vi "Untitled 2 (SubVI).vi"(6 "input cluster in":T1 {"Image Type" items=["Grayscale (U8)", "Grayscale (U16)"]; "ROI Parameters"."Size(um)" min=0 max=255 step=0.1 format="%.2f"; "ROI Parameters"."Count" min=0 max=255 step=0.1 format="%.2f"}, 7 "Variant":variant, 8 "error in (no error)":errorcluster, 9 "reference 3":refnum<vi>, 10 "reference in":refnum<vi>, 11 "Digital in":refnum<vi>) -> (0 "error out":errorcluster, 1 "input cluster out":T1 {"Image Type" items=["Grayscale (U8)", "Grayscale (U16)"]; "ROI Parameters"."Size(um)" min=0 max=255 step=0.1 format="%.2f"; "ROI Parameters"."Count" min=0 max=255 step=0.1 format="%.2f"}, 2 "Address Var":variant, 3 "Error Var":variant)   [LabVIEW 2023, in "Camera_Controller.lvlib" / "Camera_Controller.lvclass"]
uses:
  Camera_Controller.lvclass
  Camera_Controller.lvclass/Camera_Controller.ctl
  <userlib>/_OpenG.lib/lvdata/lvdata.llb/openg_variant.lvlib
  <vilib>/vision/Image Controls.llb/IMAQ Image.ctl
  typedefs/Image Type.ctl
  typedefs/typedefs.lvlib
  typedefs/ImageProcessingParameters.ctl
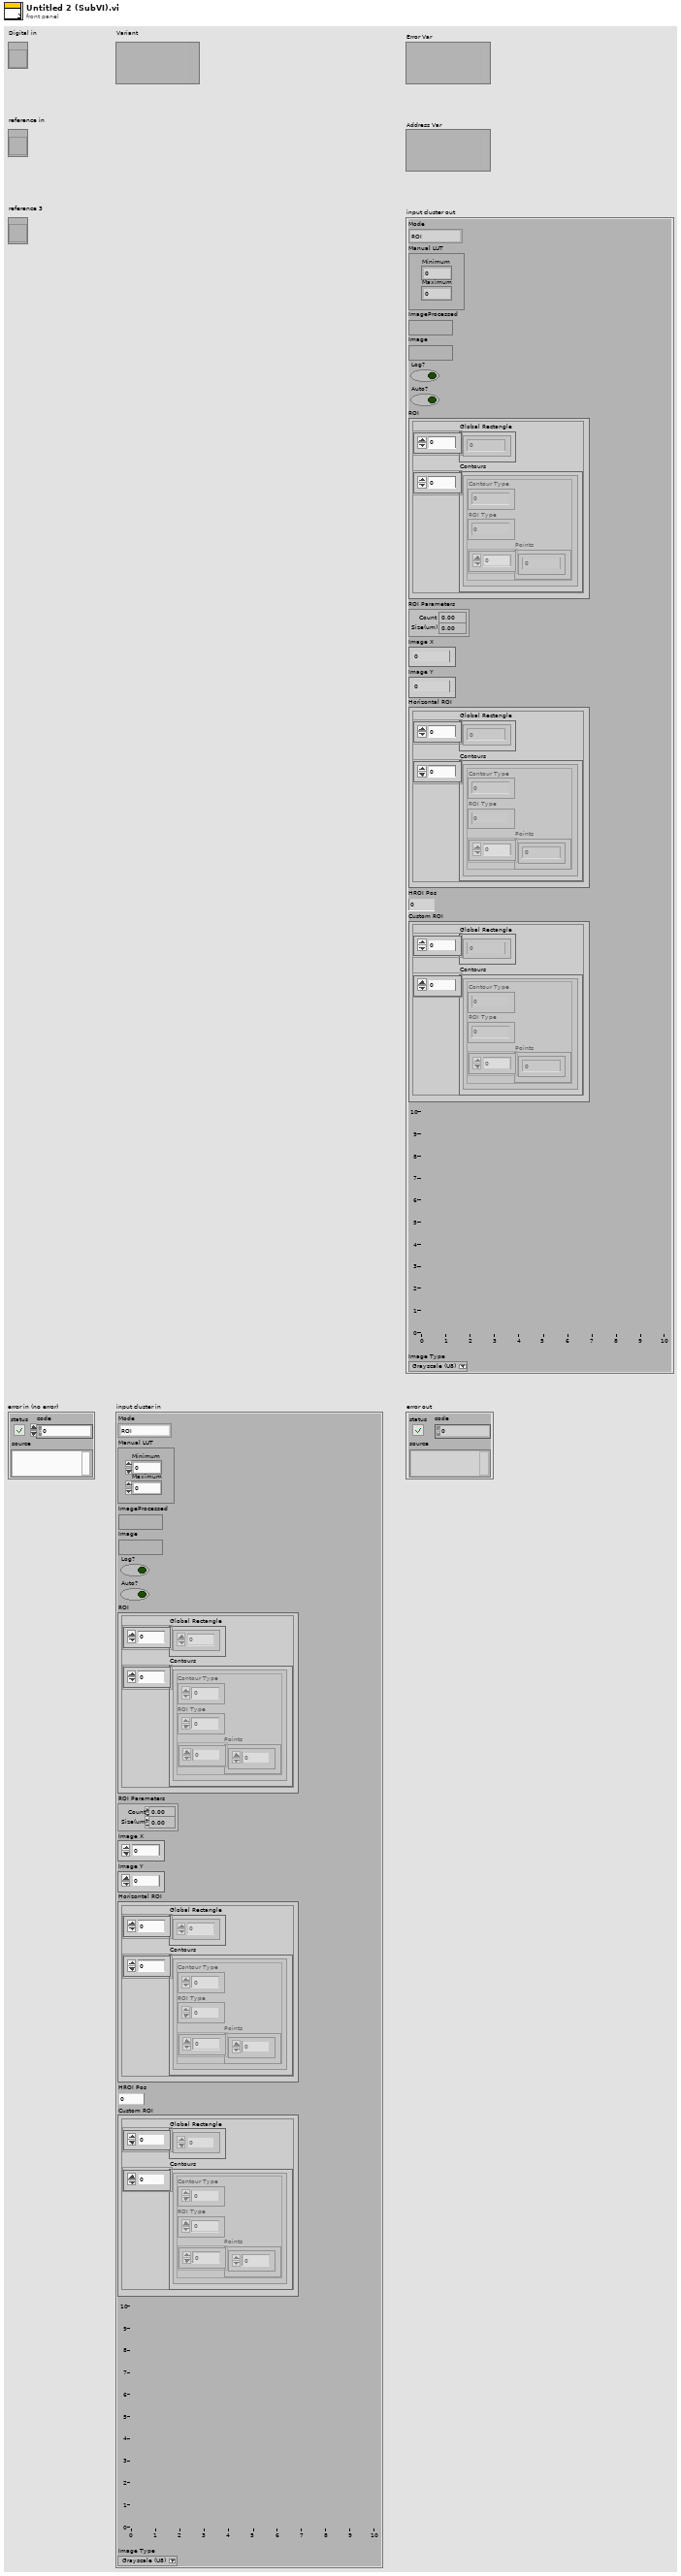
[diagram p1: front panel]
types:
  T1 = typedef "typedefs.lvlib/ImageProcessingParameters.ctl" = cluster{"Mode":enum16{"ROI", "Image"}, "Manual LUT":cluster{"Minimum":dbl, "Maximum":dbl}, "ImageProcessed":T2, "Image ":T2, "Log?":bool, "Auto?":bool, "ROI":cluster{"Global Rectangle":i32[], "Contours":cluster{"Contour Type":u32, "ROI Type":u32, "Points":i32[]}[]}, "ROI Parameters":cluster{"Count":sgl, "Size(um)":sgl}, "Image X":i32, "Image Y":i32, "Horizontal ROI":cluster{"Global Rectangle":i32[], "Contours":cluster{"Contour Type":u32, "ROI Type":u32, "Points":i32[]}[]}, "HROI Pos":u16, "Custom ROI":cluster{"Global Rectangle":i32[], "Contours":cluster{"Contour Type":u32, "ROI Type":u32, "Points":i32[]}[]}, "Intensity Graph":u8[][], "Image Type":T3}
  T2 = typedef "IMAQ Image.ctl" = refnum<image>
  T3 = typedef "typedefs.lvlib/Image Type.ctl" = u32
  T4 = typedef "Image Type" = u32
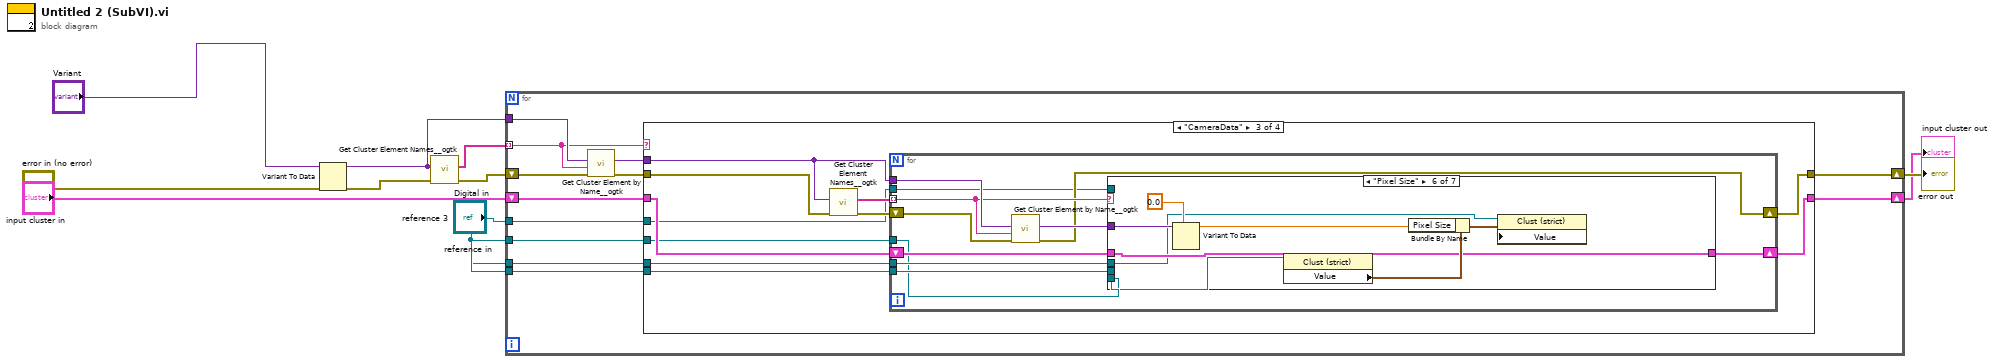
[diagram p0: block diagram]
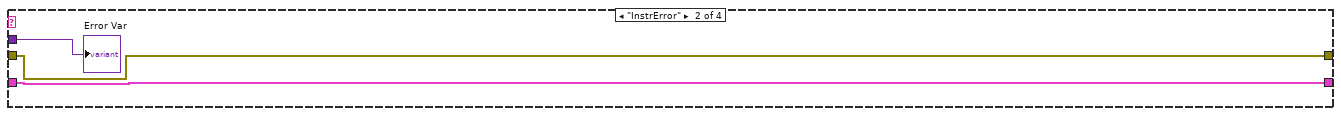
[diagram p3: hidden frame]
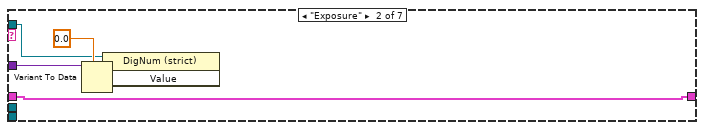
[diagram p5: hidden frame]
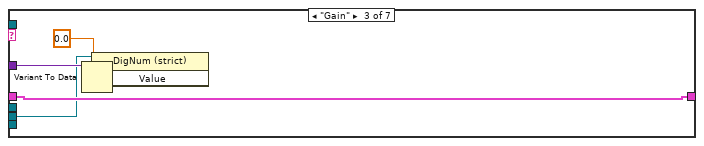
[diagram p6: hidden frame]
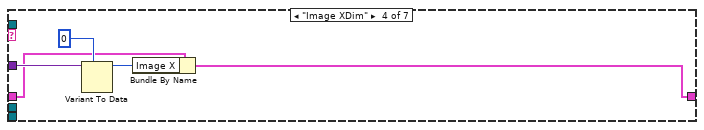
[diagram p7: hidden frame]
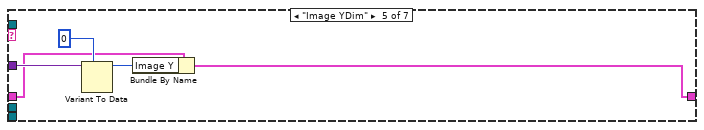
[diagram p8: hidden frame]
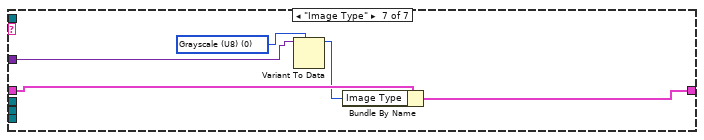
[diagram p9: hidden frame]
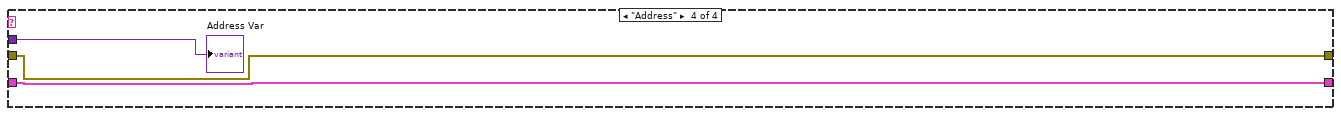
[diagram p10: hidden frame]
diagram:
  n1 = Variant To Data(error in="error in (no error)", Variant="Variant") -> (data=w7:variant, error out=w11:errorcluster)  [unwired: 1 in]
  n2 = call <userlib>:"Get Cluster Element Names__ogtk.vi"("error in (no error)"=w11, "Cluster"=w7) -> ("error out"=w10:errorcluster, "Element Names"=w6:string[])  [unwired: 8 in]
  n3 = for {
    tunnel: w6 -> [w23] mode=indexing
    tunnel: w7 -> [w24]
    shift-right: [w18] -> w12
    shift-left: w10 -> [w19]
    shift-right: [w17] -> w9
    shift-left: "input cluster in" -> [w21]
    tunnel: "Digital in" -> [w16]
    tunnel: "reference in" -> [w15]
    tunnel: "reference 3" -> [w14]
    tunnel: "reference 3" -> [w13]
    n4 = call <userlib>:"Get Cluster Element by Name__ogtk.vi"("error in (no error)"=w19, "Element Name"=w23, "Cluster"=w24) -> ("error out"=w20:errorcluster, "VElement"=w22:variant)  [unwired: 6 in, 1 out]
    n5 = case shown="\"CameraData\"" w23 {
      tunnel: w22 -> [_ w29 w39 w88]
      tunnel: w21 -> [w26 w28 w38 w87]
      tunnel: [w26 w28 w37 w87] -> w17
      tunnel: w20 -> [w25 w27 w36 w86]
      tunnel: [w25 w27 w34 w86] -> w18
      tunnel: w16 -> [_ _ w33 _]
      tunnel: w15 -> [_ _ w32 _]
      tunnel: w14 -> [_ _ w31 _]
      tunnel: w13 -> [_ _ w30 _]
      frame "False", Default {
      }
      frame "InstrError" {
        "Error Var" <- w29
      }
      frame "CameraData" {
        n6 = call <userlib>:"Get Cluster Element Names__ogtk.vi"("error in (no error)"=w36, "Cluster"=w39) -> ("error out"=w35:errorcluster, "Element Names"=w40:string[])  [unwired: 8 in]
        n7 = for {
          tunnel: w40 -> [w50] mode=indexing
          tunnel: w39 -> [w51]
          shift-right: [w45] -> w34
          shift-left: w35 -> [w46]
          shift-right: [w47] -> w37
          shift-left: w38 -> [w48]
          tunnel: w33 -> [w44]
          tunnel: w32 -> [w43]
          tunnel: w31 -> [w42]
          tunnel: w30 -> [w41]
          n8 = call <userlib>:"Get Cluster Element by Name__ogtk.vi"("error in (no error)"=w46, "Element Name"=w50, "Cluster"=w51) -> ("error out"=w45:errorcluster, "VElement"=w49:variant)  [unwired: 6 in, 1 out]
          n9 = case shown="\"Gain\"" w50 {
            tunnel: w49 -> [_ w57 w62 w67 w72 w80 w85]
            tunnel: w48 -> [w52 w54 w59 w65 w69 w75 w84]
            tunnel: [w52 w54 w59 w64 w68 w75 w83] -> w47
            tunnel: w44 -> [_ w53 _ _ _ _ _]
            tunnel: w43 -> [_ _ w58 _ _ _ _]
            tunnel: w42 -> [_ _ _ _ _ w74 _]
            tunnel: w41 -> [_ _ _ _ _ w73 _]
            frame "False", Default {
            }
            frame "Exposure" {
              n10 = Variant To Data(type=0.0, Variant=w57) -> (data=w55:dbl)  [unwired: 1 in, 1 out]
              n11 = property class="DigNum (strict)"(reference=w53, "Value"=w55) -> ()  [unwired: 1 in, 2 out]
            }
            frame "Gain" {
              n12 = Variant To Data(type=0.0, Variant=w62) -> (data=w60:dbl)  [unwired: 1 in, 1 out]
              n13 = property class="DigNum (strict)"(reference=w58, "Value"=w60) -> ()  [unwired: 1 in, 2 out]
            }
            frame "Image XDim" {
              n14 = Variant To Data(type=u16 0 ("Image XDim"), Variant=w67) -> (data=w63:u16)  [unwired: 1 in, 1 out]
              n15 = Bundle By Name(cluster=w65, "Image X"=w63) -> (w64:T1)
            }
            frame "Image YDim" {
              n16 = Variant To Data(type=u16 0 ("Image XDim"), Variant=w72) -> (data=w70:u16)  [unwired: 1 in, 1 out]
              n17 = Bundle By Name(cluster=w69, "Image Y"=w70) -> (w68:T1)
            }
            frame "Pixel Size" {
              n18 = Variant To Data(type=0.0 ("Image XDim"), Variant=w80) -> (data=w76:dbl)  [unwired: 1 in, 1 out]
              n19 = property class="Clust (strict)"(reference=w73) -> ("Value"=w77:cluster{"Pixel Size":dbl})  [unwired: 1 in, 2 out]
              n20 = Bundle By Name(cluster=w77, "Pixel Size"=w76) -> (w78:cluster{"Pixel Size":dbl})
              n21 = property class="Clust (strict)"(reference=w74, "Value"=w78) -> ()  [unwired: 1 in, 2 out]
            }
            frame "Image Type" {
              w81 = T4 0 items=["Grayscale (U8)", "Grayscale (I16)", "Grayscale (SGL)", "Complex (CSG)", "RGB (U32)", "HSL (U32)", "RGB (U64)", "Grayscale (U16)"] ("Image Type")
              n22 = Variant To Data(type=w81, Variant=w85) -> (data=w82:T4)  [unwired: 1 in, 1 out]
              n23 = Bundle By Name(cluster=w84, "Image Type"=w82) -> (w83:T1)
            }
          }
        }
      }
      frame "Address" {
        "Address Var" <- w88
      }
    }
  }
  "error out" <- w12
  "input cluster out" <- w9
